vi "niDTS WLAN INSTR TX Initiate.vi"(8 "error in (no error)":errorcluster, 9 "Result Instance":i32=1, 10 "Driver Instance":i32=1, 11 "niDTS WLAN INSTR TX in":refnum<class "niDTS WLAN INSTR TX.lvclass">) -> (0 "error out":errorcluster, 3 "niDTS WLAN INSTR TX out":refnum<class "niDTS WLAN INSTR TX.lvclass">)   [LabVIEW 2015, in "niDTS WLAN.lvlib" / "niDTS WLAN INSTR TX.lvclass"]
uses:
  niDTS WLAN INSTR TX.lvclass
  niDTS WLAN INSTR TX.lvclass/niDTS WLAN INSTR TX.ctl
  RiviInstDriver/niRfsaWlan/Objects/niRfsaWlan.lvclass
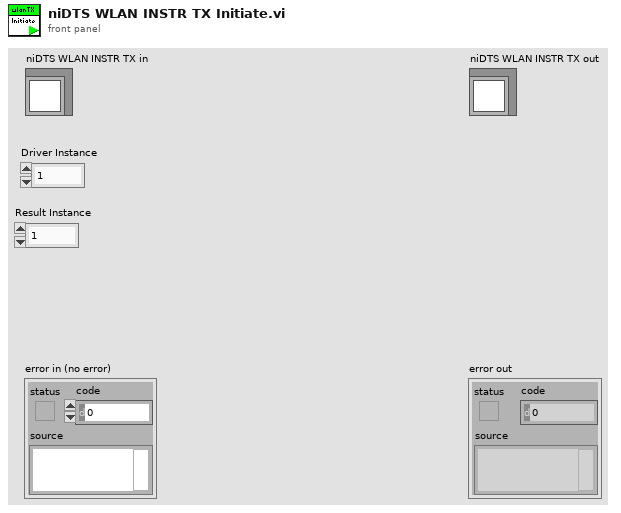
[diagram p1: front panel]
types:
  T1 = typedef "niRfsaWlan.lvclass/niRfsaWlan INC Handle.ctl" = refnum<data-value>
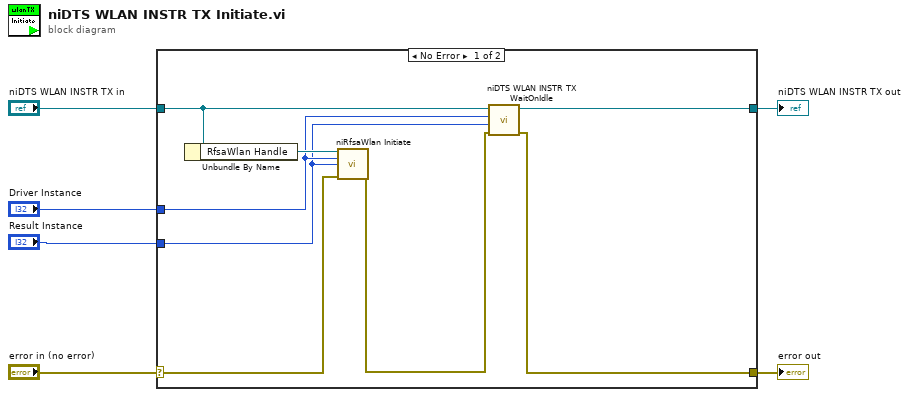
[diagram p0: block diagram]
diagram:
  n1 = case shown="No Error" "error in (no error)" {
    selector: "error in (no error)" -> [w13 w16]
    tunnel: [w9 w16] -> w5
    tunnel: [w10 w15] -> w3
    tunnel: "niDTS WLAN INSTR TX in" -> [w11 w15]
    tunnel: "Driver Instance" -> [w8 _]
    tunnel: "Result Instance" -> [w7 _]
    frame No Error {
      n2 = Unbundle By Name(w11) -> ("RfsaWlan Handle"=w14:T1)
      n3 = call "niRfsaWlan Initiate.vi"("InstDriver Handle in"=w14, "Driver Instance"=w8, "Result Instance"=w7, "error in (no error)"=w13) -> ("error out"=w12:errorcluster)  [unwired: 10 in, 1 out]
      n4 = call-dynamic "niDTS WLAN INSTR TX WaitOnIdle.vi"("error in (no error)"=w12, "Result Instance"=w7, "Driver Instance"=w8, "niDTS WLAN INSTR TX in"=w11) -> ("error out"=w9:errorcluster, "niDTS WLAN INSTR TX out"=w10:refnum<class "niDTS WLAN INSTR TX.lvclass">)  [unwired: 6 in]
    }
    frame Error {
    }
  }
  "error out" <- w5
  "niDTS WLAN INSTR TX out" <- w3
